vi "field emission sensor_dev_broken.vi"() -> ()   [LabVIEW 2014]
uses:
  Keithley 24XX/Keithley 24XX.lvlib
  <userlib>/Nanonis Prog Interface V5/Nanonis Prog Interface.lvlib
  <vilib>/Analysis/NI_AALBase.lvlib
panel:
  in  "Output Mode (0: Fixed) 2":u16(ring) items=["Fixed", "Sweep", "List"]
  in  "Sample Count (1) 2":i32=1
  in  "p Current Amplitude (A)":dbl=-0.3 format="%#_6p"
  in  "Current Amplitude Max (A)":sgl=1.5e-10 format="%#_6p"
  in  "Std threshold":dbl=5e-12 format="%#_6p"
  in  "Mean threshold":dbl=2e-11 format="%#_6p"
  out "ramp paused":bool
  out "x+y":sgl=1.4799449e-10
  out "amplitude":sgl(graph)=1.0739469e-11
  in  "Amplitude (V) (NaN=no change)":sgl=nan
  in  "Frequency (Hz) (NaN=no change)":sgl=nan format="%#_6p"
  in  "p Amplitude":dbl=-0.3 format="%#_6p"
  in  "amplitude max":sgl=1.5e-10 format="%#_6p"
  in  "Signal index (0-79)":i8=49
  out "amplitude":sgl=1.0739469e-11 format="%#_6p"
  in  "dz":dbl=1e-09 format="%#_6p"
  in  "ramp delay (s)":dbl=0.001
  out "ramp trigger":bool
  out "millisecond timer value":u32=272952714
  in  "Clear plots":bool
  out "z":dbl(graph)=7.783200430924225e-08
  in  "Ramp":bool
  in  "steps":sgl=5e-09 format="%#_6p"
  in  "Ramp to":sgl=1.3e-06 format="%#_6p"
  in  "I":sgl=5e-05 format="%#_6p"
  in  "PID":bool
  in  "p":sgl=0.01 format="%#_6p"
  in  "setpoint":sgl format="%#_3p"
  in  "max Current":sgl=2e-06 format="%#_6p"
  in  "setpoint approach":sgl=3e-08 format="%#_6p"
  in  "auto approach":bool
  in  "Number of steps":u16=1
  in  "withdraw tip":bool
  in  "coarse step":bool
  in  "Direction":enum16{"X +", "X -", "Y +", "Y -", "Z +", "Z -"}(ring)=enum."Z +"
  in  "Machine name (local machine IP)":string="localhost"
  in  "Z position [m]":dbl=7.783200430924225e-08 max=1.096e-07 step=1.0 format="%_6p"
  out "current [A]":sgl=-1.479945e-08 format="%#_6p"
  in  "time divider":dbl=60.0
  out "time elapsed":dbl=72.48559594154358
  in  "milliseconds to wait":u32=100
  in  "VISA resource name":refnum<visa-resource-name>="GPIB0::21::INSTR"
  in  "stop":bool
  in  "current multiplier":sgl=1.0
  out "Current":sgl(graph)=-1.479945e-08
  # "STOP the VI during an Nanonis Auto Approach"
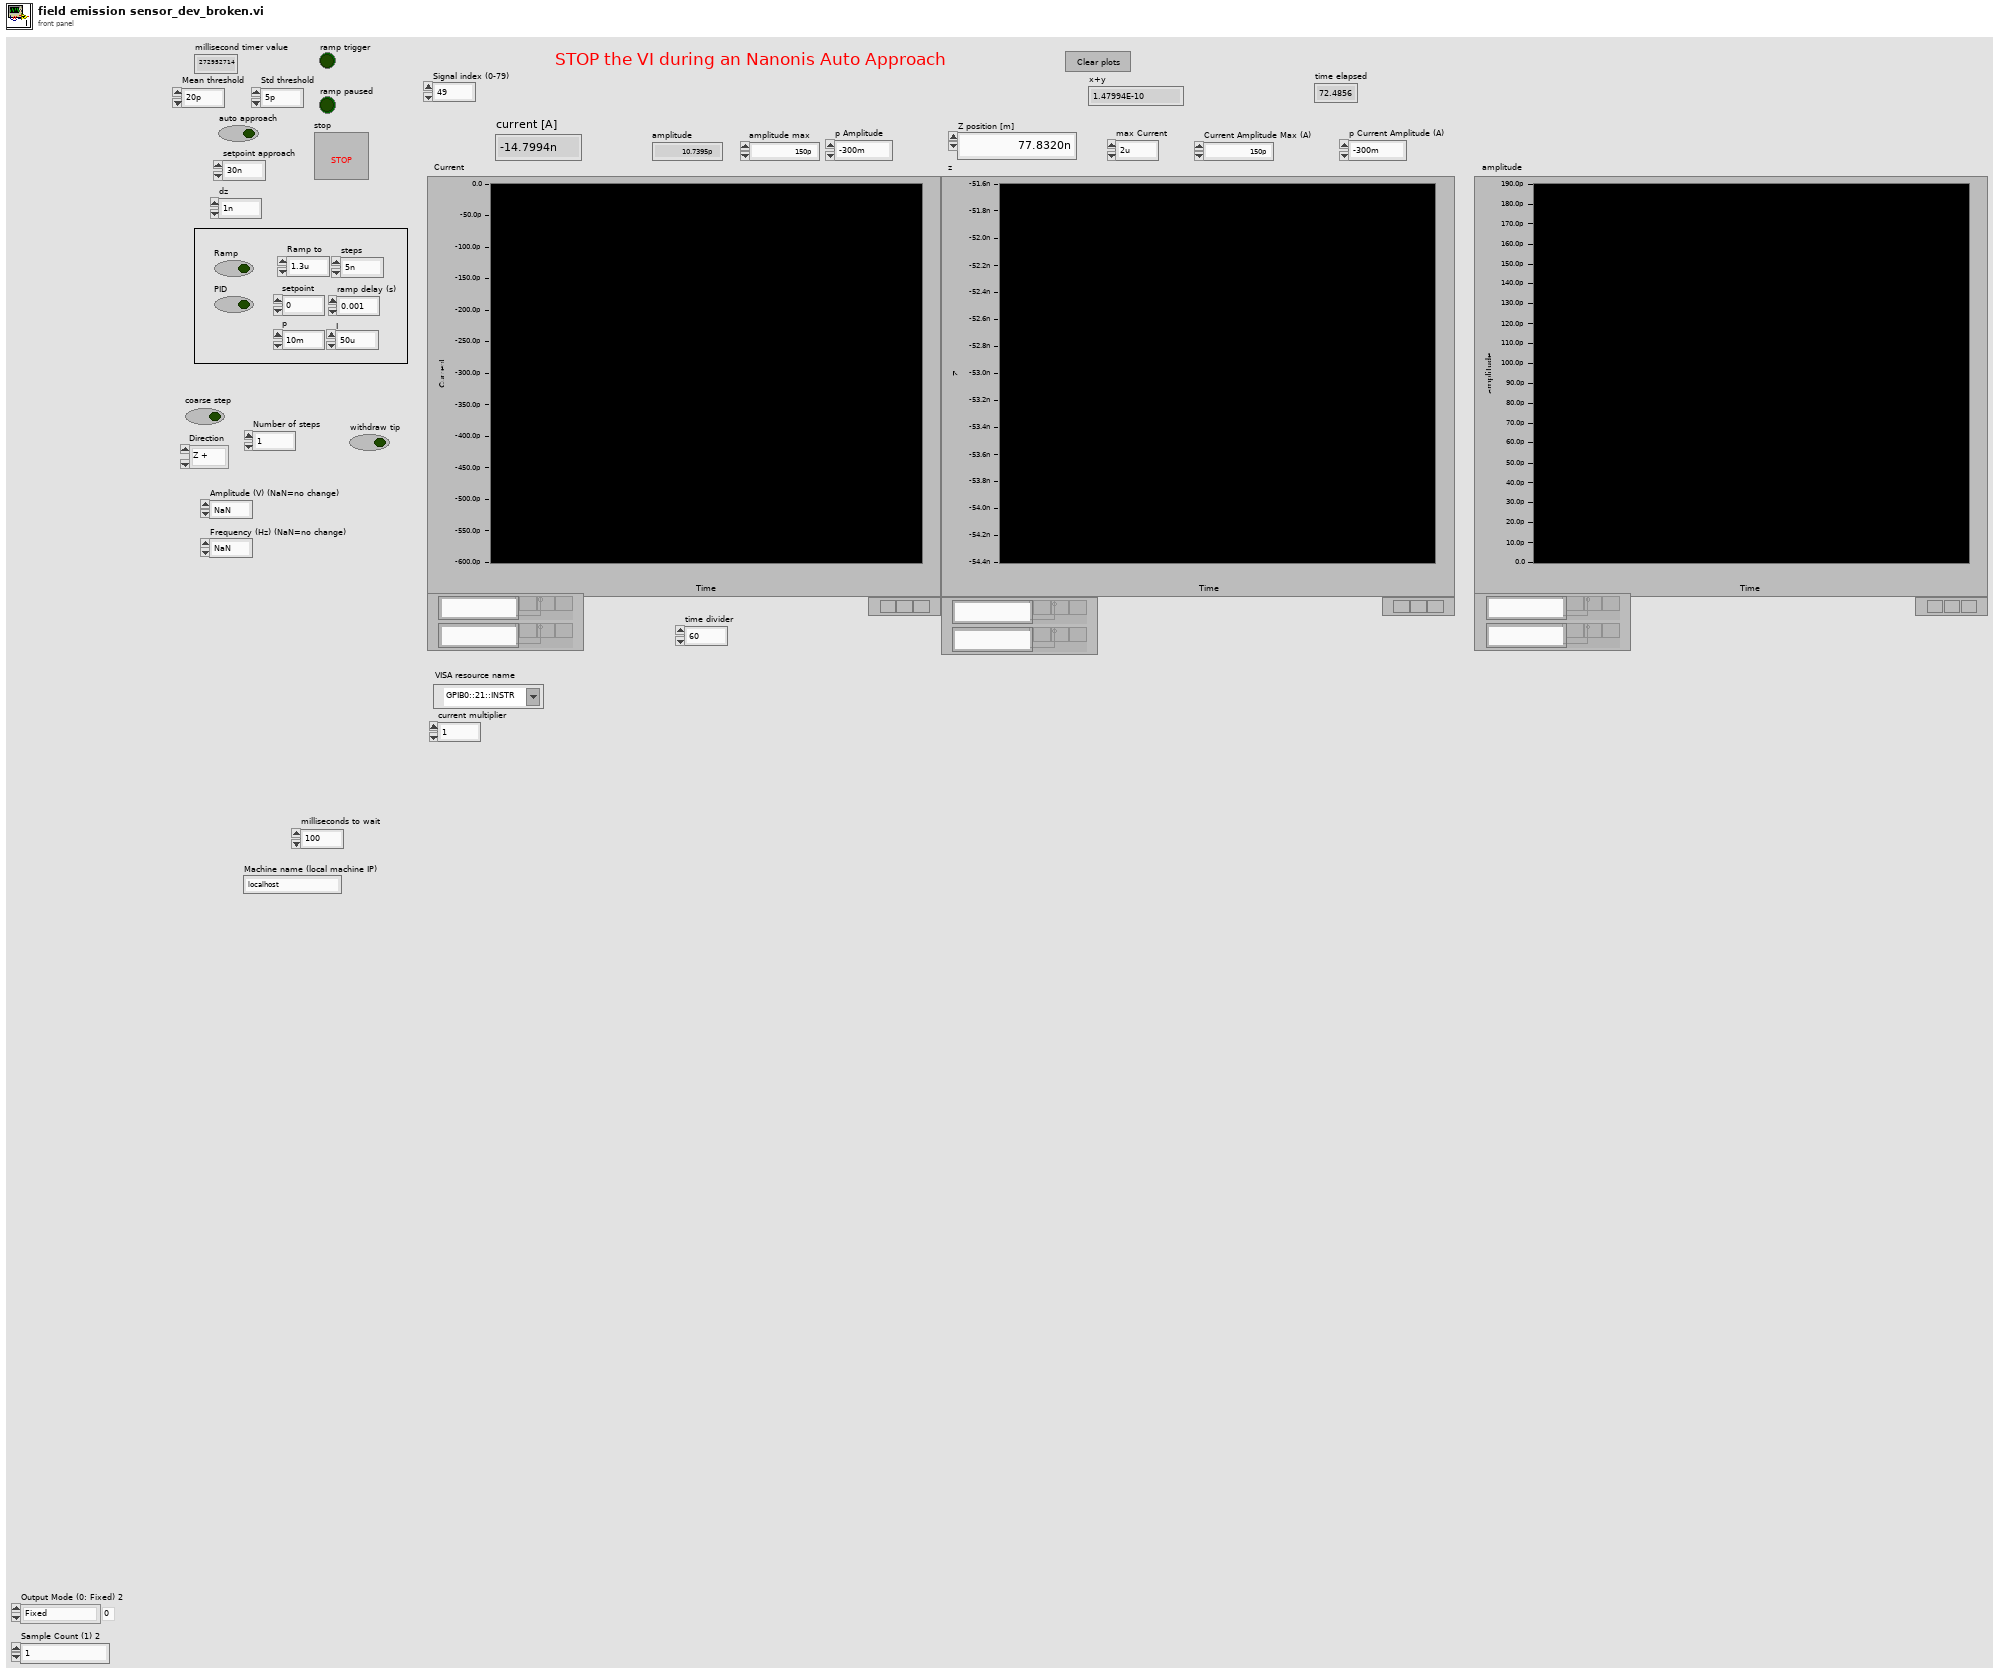
[diagram p1: front panel]
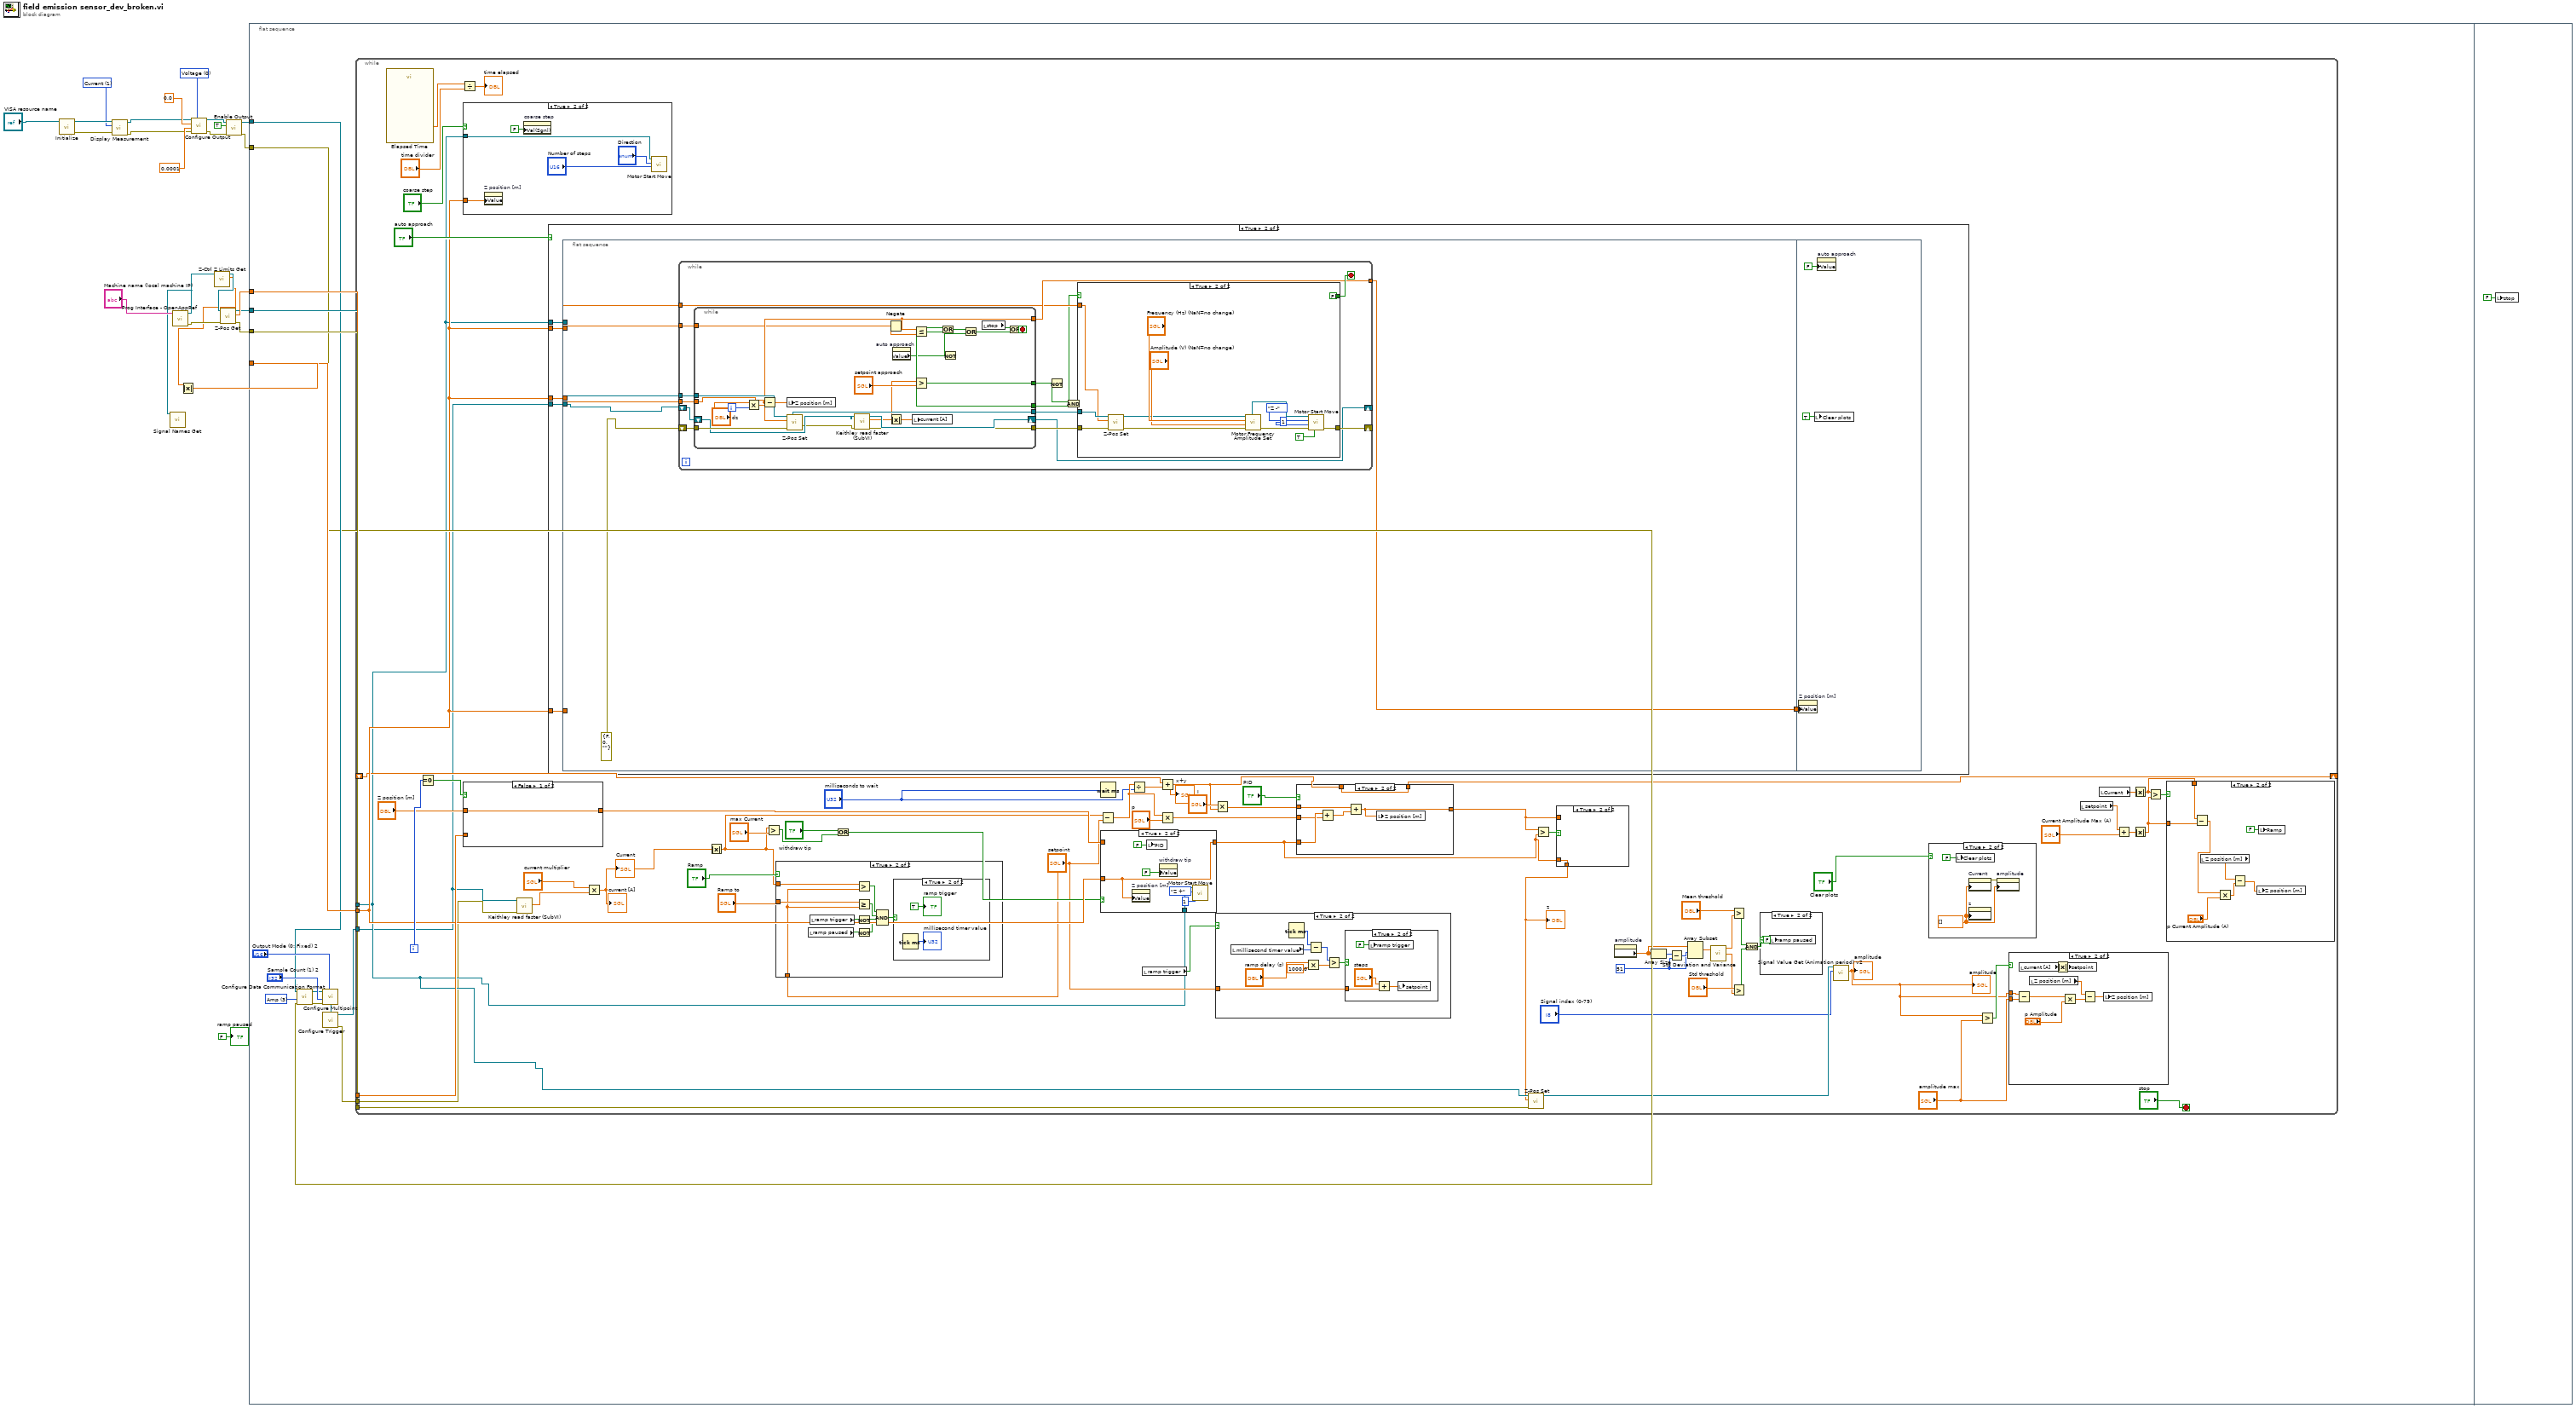
[diagram p0: block diagram]
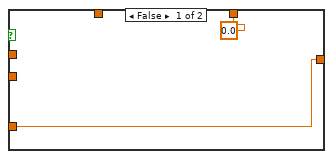
[diagram p11: hidden frame]
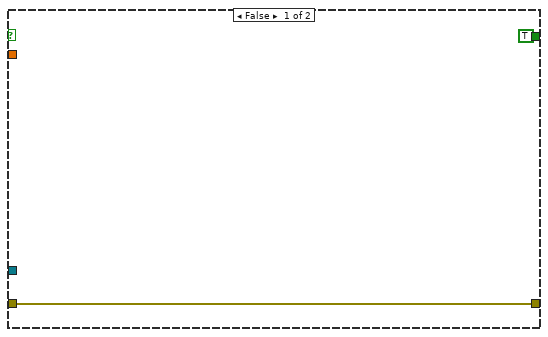
[diagram p13: hidden frame]
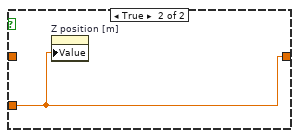
[diagram p16: hidden frame]
diagram:
  w6 = u16 1 items=["Voltage", "Current", "Resistance"] ("Displayed Measurement (0: Voltage)")
  w18 = u16 0 items=["Voltage", "Current"] ("Source Mode  (0: Voltage)")
  n1 = call "Initialize.vi"("VISA resource name"="VISA resource name") -> ("error out"=w8:errorcluster, "VISA resource name out"=w10:refnum<visa-resource-name>)  [unwired: 9 in]
  n2 = call "Display Measurement.vi"("error in (no error)"=w8, "Displayed Measurement (0: Voltage)"=w6, "VISA resource name"=w10) -> ("error out"=w7:errorcluster, "VISA resource name out"=w9:refnum<visa-resource-name>)  [unwired: 7 in]
  n3 = call <userlib>:"Prog Interface - OpenAppRef.vi"("Machine name (local machine IP)"="Machine name (local machine IP)") -> ("Error out"=w23:errorcluster, "Application reference"=w2:refnum<vi>)  [unwired: 5 in]
  n4 = call <userlib>:"Signal Names Get.vi"("Application ref in"=w2) -> ()  [unwired: 6 in, 3 out]
  n5 = call "Configure Output.vi"("Source Mode  (0: Voltage)"=w18, "error in (no error)"=w7, "Compliance  Level (0.1)"=0.0001, "Output Level (0)"=0.0, "VISA resource name"=w9) -> ("error out"=w14:errorcluster, "VISA resource name out"=w15:refnum<visa-resource-name>)  [unwired: 5 in]
  n6 = call <userlib>:"Z-Ctrl Z Limits Get.vi"("Application ref in"=w2) -> ("Z high limit"=w3:sgl, "Application ref out"=w4:refnum<vi>)  [unwired: 7 in, 2 out]
  n7 = Absolute Value(x=w3) -> (abs(x)=w5:sgl)
  n8 = call <userlib>:"Z-Pos Get.vi"("error in (no error)"=w23, "Application ref in"=w4) -> ("error out"=w22:errorcluster, "Z position (m)"=w21:sgl, "Application ref out"=w20:refnum<vi>)  [unwired: 7 in]
  n9 = call "Enable Output.vi"("error in (no error)"=w14, "Enable Output (T: Enable)"=TRUE, "VISA resource name"=w15) -> ("error out"=w11:errorcluster, "VISA resource name out"=w12:refnum<visa-resource-name>)  [unwired: 7 in]
  n10 = flat-sequence {
    tunnel: w22 -> [w39]
    tunnel: w21 -> [w38]
    tunnel: w20 -> [w37]
    tunnel: w12 -> [w28]
    tunnel: w11 -> [w25]
    tunnel: w5 -> [w36]
    frame #0 {
      w35 = u16 3 items=["All", "Volt and Amp", "Volt", "Amp"] ("Data Selection (0: All)")
      n11 = call "Configure Data Communication Format.vi"("error in (no error)"=w25, "Data Selection (0: All)"=w35, "VISA resource name"=w28) -> ("error out"=w29:errorcluster, "VISA resource name out"=w30:refnum<visa-resource-name>)  [unwired: 7 in]
      n12 = call "Configure Multipoint.vi"("Output Mode (0: Fixed)"="Output Mode (0: Fixed) 2", "error in (no error)"=w29, "Trigger Count (1)"="Sample Count (1) 2", "VISA resource name"=w30) -> ("error out"=w33:errorcluster, "VISA resource name out"=w34:refnum<visa-resource-name>)  [unwired: 6 in]
      n13 = call "Configure Trigger.vi"("error in (no error)"=w33, "VISA resource name"=w34) -> ("error out"=w26:errorcluster, "VISA resource name out"=w27:refnum<visa-resource-name>)  [unwired: 8 in]
      n14 = while {
        tunnel: w37 -> [w66]
        tunnel: w39 -> [w103]
        tunnel: w38 -> [w102]
        tunnel: w27 -> [w40]
        tunnel: w26 -> [w41]
        tunnel: w36 -> [w93]
        shift-right: [w78] -> _
        shift-left: _ -> [w85]
        i -> [w101]
        stop <- "stop" stop-if-true
        w58 = 51 ("y")
        n15 = call "Elapsed Time"() -> ("Elapsed Time (s)"=w104:dbl)  [unwired: 12 in, 7 out]
        n16 = Equal To 0?(x=w101) -> (x = 0?=w100:bool)
        n17 = Divide(x=w104, y="time divider") -> (x/y=→"time elapsed":dbl)
        n18 = case shown="True" "coarse step" {
          tunnel: w66 -> [_ w247]
          tunnel: w93 -> [_ w243]
          frame False {
          }
          frame True {
            n19 = property on="Z position [m]" class="DigNum (strict)"("Value"=w243) -> ()  [unwired: 2 in, 2 out]
            n20 = property on="coarse step" class="Bool (strict)"("Val(Sgnl)"=FALSE ("Value (Signaling)")) -> ()  [unwired: 2 in, 2 out]
            n21 = call <userlib>:"Motor Start Move.vi"("Number of steps"="Number of steps", "Direction"="Direction", "Application ref in"=w247) -> ()  [unwired: 6 in, 2 out]
          }
        }
        n22 = case shown="False" w100 {
          tunnel: [w248 w249] -> w97
          tunnel: w102 -> [_ w249]
          tunnel: "Z position [m]" -> [w248 _]
          frame False {
          }
          frame True {
            n23 = property on="Z position [m]" class="DigNum (strict)"("Value"=w249) -> ()  [unwired: 2 in, 2 out]
          }
        }
        n24 = call "Keithley read faster (SubVI).vi"("error in (no error)"=w41, "VISA Refnum in"=w40) -> ("Numeric"=w42:sgl)  [unwired: 7 in, 2 out]
        n25 = case shown="True" "auto approach" {
          tunnel: w40 -> [_ w168]
          tunnel: w66 -> [_ w167]
          tunnel: w93 -> [_ w165]
          tunnel: w93 -> [_ w164]
          tunnel: w93 -> [_ w163]
          frame False {
          }
          frame True {
            n26 = flat-sequence {
              tunnel: w168 -> [w169]
              tunnel: w167 -> [w175]
              tunnel: [w174] -> w166
              tunnel: w165 -> [w173]
              tunnel: w164 -> [w172]
              tunnel: w163 -> [w171]
              tunnel: w166 -> [w234]
              frame #0 {
                n27 = while {
                  tunnel: w175 -> [w190]
                  tunnel: [w184] -> w174
                  tunnel: w173 -> [w183]
                  tunnel: w172 -> [w182]
                  tunnel: w171 -> [w181]
                  shift-right: [w180] -> _
                  shift-left: errorcluster {"status"=FALSE, "code"=0, "source"=""} ("error in (no error)") -> [w179]
                  shift-right: [w176] -> _
                  shift-left: w169 -> [w191]
                  stop <- w185 stop-if-true
                  n28 = while {
                    tunnel: w190 -> [w231]
                    tunnel: [w230] -> w189
                    tunnel: [w229] -> w188
                    tunnel: [w228] -> w187
                    tunnel: [w210] -> w186
                    tunnel: [w227] -> w184
                    tunnel: w183 -> [w226]
                    tunnel: w181 -> [w224]
                    tunnel: w179 -> [w213]
                    shift-right: [w211] -> w176
                    shift-left: w191 -> [w212]
                    i -> [w232]
                    stop <- w219 stop-if-true
                    n29 = Multiply(x="dz", y=w232) -> (x*y=w215:dbl)
                    n30 = Subtract(x=w226, y=w215) -> (x-y=w227:dbl)
                    n31 = local write "Z position [m]"(w227) -> ()
                    n32 = call <userlib>:"Z-Pos Set.vi"("error in (no error)"=w213, "Z position (m)"=w227, "Application ref in"=w231) -> ("error out"=w209:errorcluster, "Application ref out"=w228:refnum<vi>)  [unwired: 7 in]
                    n33 = call "Keithley read faster (SubVI).vi"("error in (no error)"=w209, "VISA Refnum in"=w212) -> ("error out"=w210:errorcluster, "Numeric"=w208:sgl, "VISA Refnum out"=w211:refnum<visa-resource-name>)  [unwired: 7 in]
                    n34 = Negate(x=w224) -> (-x=w225:sgl)
                    n35 = Absolute Value(x=w208) -> (abs(x)=w216:sgl)
                    n36 = property on="auto approach" class="Bool (strict)"() -> ("Value"=w222:bool)  [unwired: 2 in, 2 out]
                    n37 = local write "current [A]"(w216) -> ()
                    n38 = Less Or Equal?(x=w227, y=w225) -> (x <= y?=w229:bool)
                    n39 = Greater?(x=w216, y="setpoint approach") -> (0:w230:bool)
                    n40 = Or(x=w230, y=w229) -> (x .or. y?=w223:bool)
                    n41 = Not(x=w222) -> (.not. x?=w221:bool)
                    n42 = Or(x=w223, y=w221) -> (x .or. y?=w220:bool)
                    n43 = local read "stop"() -> (w218:bool)
                    n44 = Or(x=w218, y=w220) -> (x .or. y?=w219:bool)
                  }
                  n45 = Not(x=w189) -> (.not. x?=w178:bool)
                  n46 = And(x=w178, y=w188) -> (x .and. y?=w177:bool)
                  n47 = case shown="True" w177 {
                    tunnel: w187 -> [_ w207]
                    tunnel: w186 -> [w192 w206]
                    tunnel: [TRUE FALSE] -> w185
                    tunnel: w182 -> [_ w202]
                    tunnel: [w192 w195] -> w180
                    frame False {
                    }
                    frame True {
                      n48 = call <userlib>:"Z-Pos Set.vi"("error in (no error)"=w206, "Z position (m)"=w202, "Application ref in"=w207) -> ("error out"=w199:errorcluster, "Application ref out"=w194:refnum<vi>)  [unwired: 7 in]
                      n49 = call <userlib>:"Motor Frequency Amplitude Set.vi"("Error in (no error)"=w199, "Amplitude (V) (NaN=no change)"="Amplitude (V) (NaN=no change)", "Frequency (Hz) (NaN=no change)"="Frequency (Hz) (NaN=no change)", "Application ref in"=w194) -> ("Error out"=w198:errorcluster, "Application ref out"=w200:refnum<vi>)  [unwired: 6 in]
                      n50 = call <userlib>:"Motor Start Move.vi"("Wait until finished? (F)"=TRUE, "Error in (no error)"=w198, "Number of steps"=u16 1, "Direction"=enum16{"X +", "X -", "Y +", "Y -", "Z +", "Z -"}."Z -", "Application ref in"=w200) -> ("Error out"=w195:errorcluster)  [unwired: 4 in, 1 out]
                    }
                  }
                }
              }
              frame #1 {
                n51 = property on="Z position [m]" class="DigNum (strict)"("Value"=w234) -> ()  [unwired: 2 in, 2 out]
                n52 = local write "Clear plots"(TRUE ("Clear plots")) -> ()
                n53 = property on="auto approach" class="Bool (strict)"("Value"=FALSE ("auto approach")) -> ()  [unwired: 2 in, 2 out]
              }
            }
          }
        }
        n54 = Multiply(x="current multiplier", y=w42) -> (x*y=w92:sgl)
        "Current" <- w92
        "current [A]" <- w92
        n55 = Absolute Value(x=w92) -> (abs(x)=w76:sgl)
        n56 = Greater?(x=w76, y="max Current") -> (0:w89:bool)
        n57 = case shown="True" "Ramp" {
          tunnel: w76 -> [_ w152]
          tunnel: "setpoint" -> [_ w149]
          tunnel: "Ramp to" -> [_ w150]
          frame False {
          }
          frame True {
            n58 = local read "ramp paused"() -> (w144:bool)
            n59 = local read "ramp trigger"() -> (w146:bool)
            n60 = Greater?(x=w152, y=w149) -> (0:w151:bool)
            n61 = Greater Or Equal?(x=w150, y=w149) -> (x >= y?=w147:bool)
            n62 = Not(x=w146) -> (.not. x?=w145:bool)
            n63 = Not(x=w144) -> (.not. x?=w143:bool)
            n64 = Compound Arithmetic op=AND(w151, w147, w145, w143) -> (w148:bool)
            n65 = case shown="True" w148 {
              frame False {
              }
              frame True {
                n66 = Tick Count (ms)() -> (millisecond timer value=→"millisecond timer value":u32)
                "ramp trigger" <- TRUE ("ramp")
              }
            }
          }
        }
        n67 = Or(x="withdraw tip", y=w89) -> (x .or. y?=w90:bool)
        n68 = Subtract(x=w76, y="setpoint") -> (x-y=w81:sgl)
        n69 = Wait (ms)(milliseconds to wait="milliseconds to wait") -> ()  [unwired: 1 out]
        n70 = case shown="True" w90 {
          tunnel: [w236 w241] -> w62
          tunnel: w97 -> [w236 _]
          tunnel: w93 -> [_ w241]
          tunnel: w66 -> [_ w239]
          frame False {
          }
          frame True {
            n71 = property on="Z position [m]" class="DigNum (strict)"("Value"=w241) -> ()  [unwired: 2 in, 2 out]
            n72 = local write "PID"(FALSE ("PID")) -> ()
            n73 = property on="withdraw tip" class="Bool (strict)"("Value"=FALSE ("withdraw tip")) -> ()  [unwired: 2 in, 2 out]
            n74 = call <userlib>:"Motor Start Move.vi"("Number of steps"=u16 1, "Direction"=enum16{"X +", "X -", "Y +", "Y -", "Z +", "Z -"}."Z +", "Application ref in"=w239) -> ()  [unwired: 6 in, 2 out]
          }
        }
        n75 = Divide(x=w81, y="milliseconds to wait") -> (x/y=w82:sgl)
        n76 = local read "ramp trigger"() -> (w72:bool)
        n77 = Add(x=w85, y=w82) -> (x+y=w79:sgl)
        "x+y" <- w79
        n78 = Multiply(x=w81, y="p") -> (x*y=w86:sgl)
        n79 = Multiply(x="I", y=w79) -> (x*y=w83:sgl)
        n80 = case shown="True" w72 {
          tunnel: "setpoint" -> [_ w131]
          frame False {
          }
          frame True {
            n81 = local read "millisecond timer value"() -> (w134:u32)
            n82 = Tick Count (ms)() -> (millisecond timer value=w135:u32)
            n83 = Multiply(x="ramp delay (s)", y=1000.0) -> (x*y=w128:dbl)
            n84 = Subtract(x=w135, y=w134) -> (x-y=w133:u32)
            n85 = Greater?(x=w133, y=w128) -> (0:w132:bool)
            n86 = case shown="True" w132 {
              tunnel: w131 -> [_ w137]
              frame False {
              }
              frame True {
                n87 = local write "ramp trigger"(FALSE ("ramp")) -> ()
                n88 = Add(x="steps", y=w137) -> (x+y=w139:sgl)
                n89 = local write "setpoint"(w139) -> ()
              }
            }
          }
        }
        n90 = case shown="True" "PID" {
          tunnel: w62 -> [w156 w162]
          tunnel: [w156 w158] -> w64
          tunnel: w86 -> [_ w161]
          tunnel: w83 -> [_ w159]
          tunnel: w79 -> [_ w157]
          tunnel: [sgl 0.0 w157] -> w78
          frame False {
          }
          frame True {
            n91 = Add(x=w162, y=w161) -> (x+y=w160:dbl)
            n92 = Add(x=w159, y=w160) -> (x+y=w158:dbl)
            n93 = local write "Z position [m]"(w158) -> ()
          }
        }
        n94 = Greater?(x=w64, y=w62) -> (0:w65:bool)
        n95 = case shown="True" w65 {
          tunnel: w64 -> [w117 _]
          tunnel: [w117 w118] -> w63
          tunnel: w62 -> [_ w118]
          frame False {
          }
          frame True {
          }
        }
        "z" <- w63
        n96 = call <userlib>:"Z-Pos Set.vi"("error in (no error)"=w103, "Z position (m)"=w63, "Application ref in"=w66) -> ("Application ref out"=w71:refnum<vi>)  [unwired: 7 in, 1 out]
        n97 = property on="amplitude" class="WFChart (strict)"() -> ("History Data"=w61:sgl[])  [unwired: 2 in, 2 out]
        n98 = Array Size(array=w61) -> (size(s)=w60:i32)
        n99 = Subtract(x=w60, y=w58) -> (x-y=w59:i32)
        n100 = Array Subset(array=w61, index=w59, length=w58) -> (w57:sgl[])
        n101 = call <vilib>:"Std Deviation and Variance.vi"("X"=w57) -> ("mean"=w56:dbl, "standard deviation"=w50:dbl)  [unwired: 1 in, 1 out]
        n102 = Greater?(x="Mean threshold", y=w56) -> (0:w52:bool)
        n103 = Greater?(x="Std threshold", y=w50) -> (0:w53:bool)
        n104 = And(x=w52, y=w53) -> (x .and. y?=w51:bool)
        n105 = case shown="True" w51 {
          frame False {
          }
          frame True {
            n106 = local write "ramp paused"(FALSE ("ramp paused")) -> ()
          }
        }
        n107 = call <userlib>:"Signal Value Get (Animation period) v2.vi"("Signal index (0-79)"="Signal index (0-79)", "Application ref in"=w71) -> ("Signal value"=w68:sgl)  [unwired: 6 in, 2 out]
        "amplitude" <- w68
        "amplitude" <- w68
        n108 = case shown="True" "Clear plots" {
          frame False {
          }
          frame True {
            w140 = dbl[] [] ("History Data")
            n109 = local write "Clear plots"(FALSE ("Clear plots")) -> ()
            n110 = property on="Current" class="WFChart (strict)"("History Data"=w140) -> (error out=w141:errorcluster)  [unwired: 2 in, 1 out]
            n111 = property on="z" class="WFChart (strict)"("History Data"=w140) -> ()  [unwired: 2 in, 2 out]
            n112 = property on="amplitude" class="WFChart (strict)"(error in=w141, "History Data"=w140) -> ()  [unwired: 1 in, 2 out]
          }
        }
        n113 = Greater?(x=w68, y="amplitude max") -> (0:w69:bool)
        n114 = case shown="True" w69 {
          tunnel: w68 -> [_ w125]
          tunnel: "amplitude max" -> [_ w124]
          frame False {
          }
          frame True {
            n115 = Subtract(x=w125, y=w124) -> (x-y=w123:sgl)
            n116 = local read "current [A]"() -> (w120:sgl)
            n117 = local read "Z position [m]"() -> (w127:dbl)
            n118 = Absolute Value(x=w120) -> (abs(x)=w119:sgl)
            n119 = Multiply(x=w123, y="p Amplitude") -> (x*y=w121:dbl)
            n120 = local write "setpoint"(w119) -> ()
            n121 = Subtract(x=w127, y=w121) -> (x-y=w126:dbl)
            n122 = local write "Z position [m]"(w126) -> ()
          }
        }
        n123 = local read "setpoint"() -> (w46:sgl)
        n124 = local read "Current"() -> (w45:sgl)
        n125 = Add(x=w46, y="Current Amplitude Max (A)") -> (x+y=w48:sgl)
        n126 = Absolute Value(x=w45) -> (abs(x)=w44:sgl)
        n127 = Absolute Value(x=w48) -> (abs(x)=w43:sgl)
        n128 = Greater?(x=w44, y=w43) -> (0:w47:bool)
        n129 = case shown="True" w47 {
          tunnel: w44 -> [_ w114]
          tunnel: w43 -> [_ w112]
          frame False {
          }
          frame True {
            n130 = Subtract(x=w114, y=w112) -> (x-y=w113:sgl)
            n131 = local read "Z position [m]"() -> (w110:dbl)
            n132 = Multiply(x=w113, y="p Current Amplitude (A)") -> (x*y=w111:dbl)
            n133 = Subtract(x=w110, y=w111) -> (x-y=w109:dbl)
            n134 = local write "Z position [m]"(w109) -> ()
            n135 = local write "Ramp"(FALSE ("Ramp")) -> ()
          }
        }
      }
    }
    frame #1 {
      n136 = local write "stop"(FALSE ("stop")) -> ()
    }
  }
  "ramp paused" <- FALSE ("ramp paused")
